vi "TempAcqSubVI.vi"(8 "error in (no error)":errorcluster, 11 "Data Cluster in":T1) -> (0 "error out":errorcluster, 2 "Temperature":dbl, 3 "Data Cluster out":T1)   [LabVIEW 2017]
uses:
  Controls/ShiftRegisterCluster.ctl
  <vilib>/DAQmx/read.llb/DAQmx Read (Analog DBL 1Chan 1Samp).vi
  <vilib>/DAQmx/miscellaneous.llb/DAQmx Fill In Error Info.vi
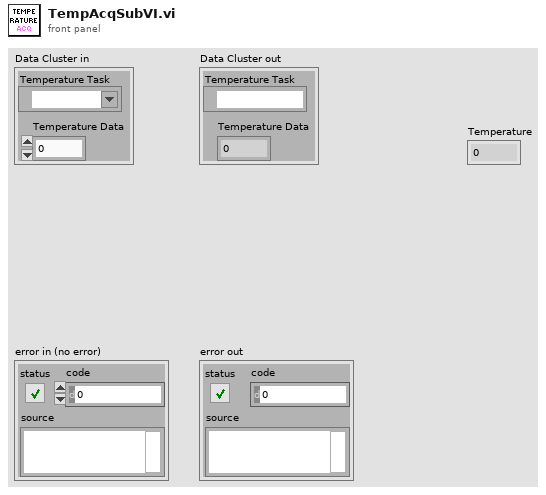
[diagram p1: front panel]
types:
  T1 = typedef "ShiftRegisterCluster.ctl" = cluster{"Temperature Task":refnum<k21>, "Temperature Data":dbl}
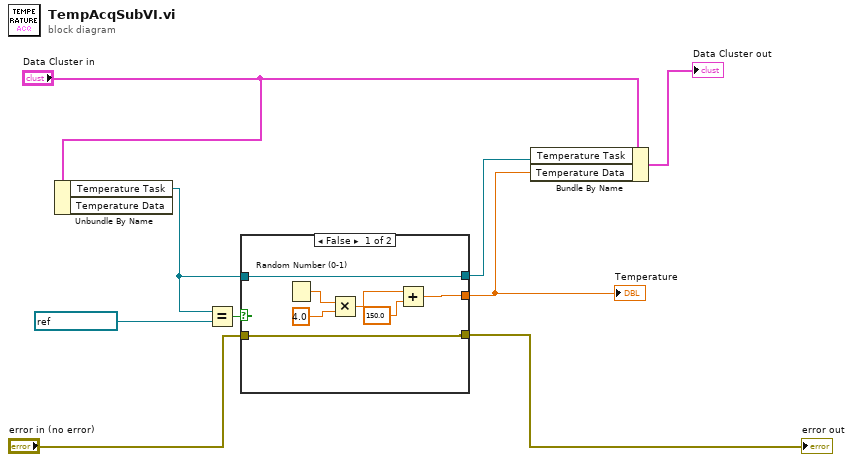
[diagram p0: block diagram]
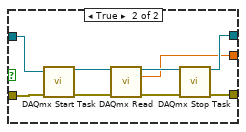
[diagram p2: hidden frame]
diagram:
  n1 = Unbundle By Name("Data Cluster in") -> ("Temperature Task"=w2:refnum<k21>)  [unwired: 1 out]
  n2 = Equal?(x=w2, y=refnum<k21> "TempTask") -> (x = y?=w3:bool)
  n3 = case shown="False" w3 {
    tunnel: [w16 w25] -> w8
    tunnel: [w13 w24] -> w6
    tunnel: "error in (no error)" -> [w13 w23]
    tunnel: w2 -> [w16 w18]
    tunnel: [w10 w17] -> w1
    frame False {
      n4 = Random Number (0-1)() -> (number: 0 to 1=w15:dbl)
      n5 = Multiply(x=w15, y=4.0) -> (x*y=w12:dbl)
      n6 = Add(x=w12, y=150.0) -> (x+y=w10:dbl)
    }
    frame True {
      n7 = call <vilib>:"DAQmx Start Task.vi"("task/channels in"=w18, "error in"=w23) -> ("task out"=w22:refnum<k21>, "error out"=w21:errorcluster)  [unwired: 12 in]
      n8 = call-poly <vilib>:"DAQmx Read.vi"("task/channels in"=w22, "error in"=w21) -> ("task out"=w20:refnum<k21>, "data"=w17:dbl, "error out"=w19:errorcluster)  [unwired: 11 in]
      n9 = call <vilib>:"DAQmx Stop Task.vi"("task/channels in"=w20, "error in"=w19) -> ("task out"=w25:refnum<k21>, "error out"=w24:errorcluster)  [unwired: 12 in]
    }
  }
  "error out" <- w6
  "Temperature" <- w1
  n10 = Bundle By Name(cluster="Data Cluster in", "Temperature Task"=w8, "Temperature Data"=w1) -> (→"Data Cluster out":T1)
